vi "테승트.vi"() -> ()   [LabVIEW 2014]
uses:
  <vilib>/httpClient/LabVIEWHTTPClient.lvlib
panel:
  out "x fmc 플랜":string caption="본문"
  out "x fmc 다운로드 주소":string caption="화이트 스페이스가 제거된 문자열"
  out "trimmed string 4":string caption="화이트 스페이스가 제거된 문자열"
  out "body 2":string caption="본문"
  out "trimmed string 3":string caption="화이트 스페이스가 제거된 문자열"
  out "FMS  주소":string
  out "FMS 플랜":string caption="본문"
  out "trimmed string 2":string caption="화이트 스페이스가 제거된 문자열"
  out "trimmed string":string caption="화이트 스페이스가 제거된 문자열"
  in  "Destination":string
  in  "departure":string
  out "?":string
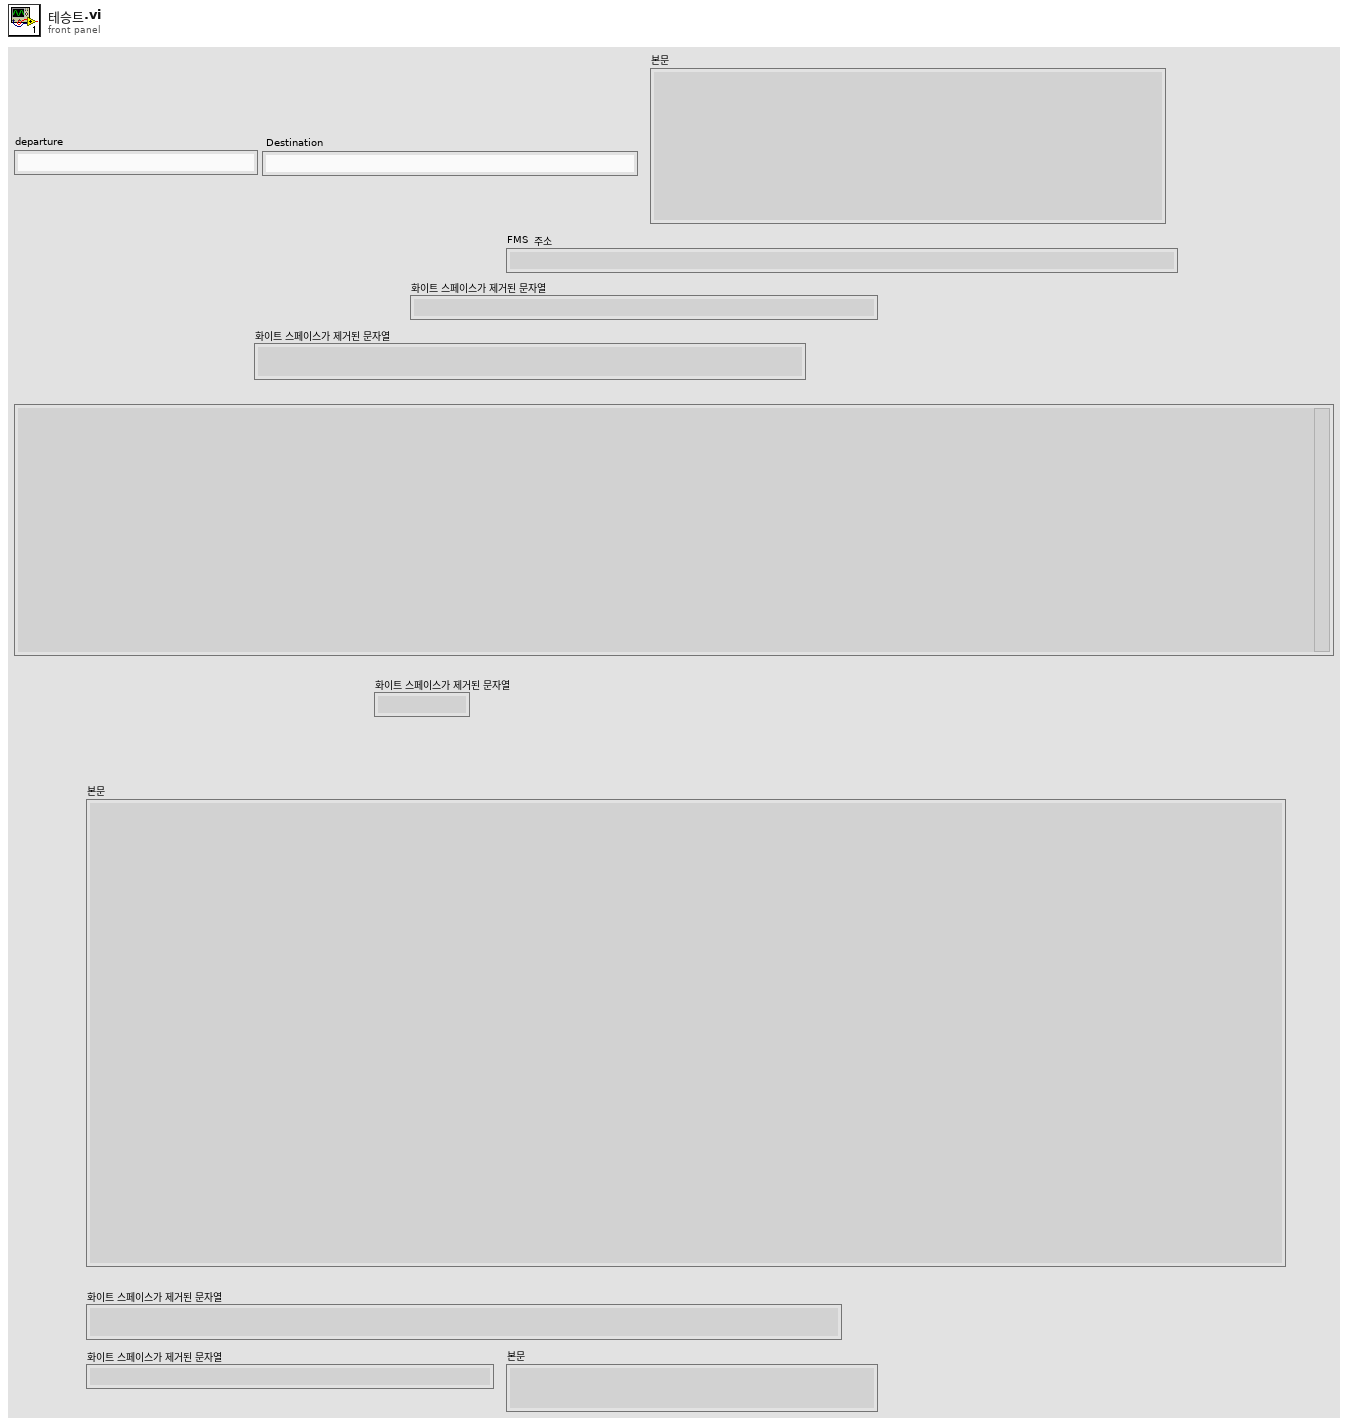
[diagram p1: front panel]
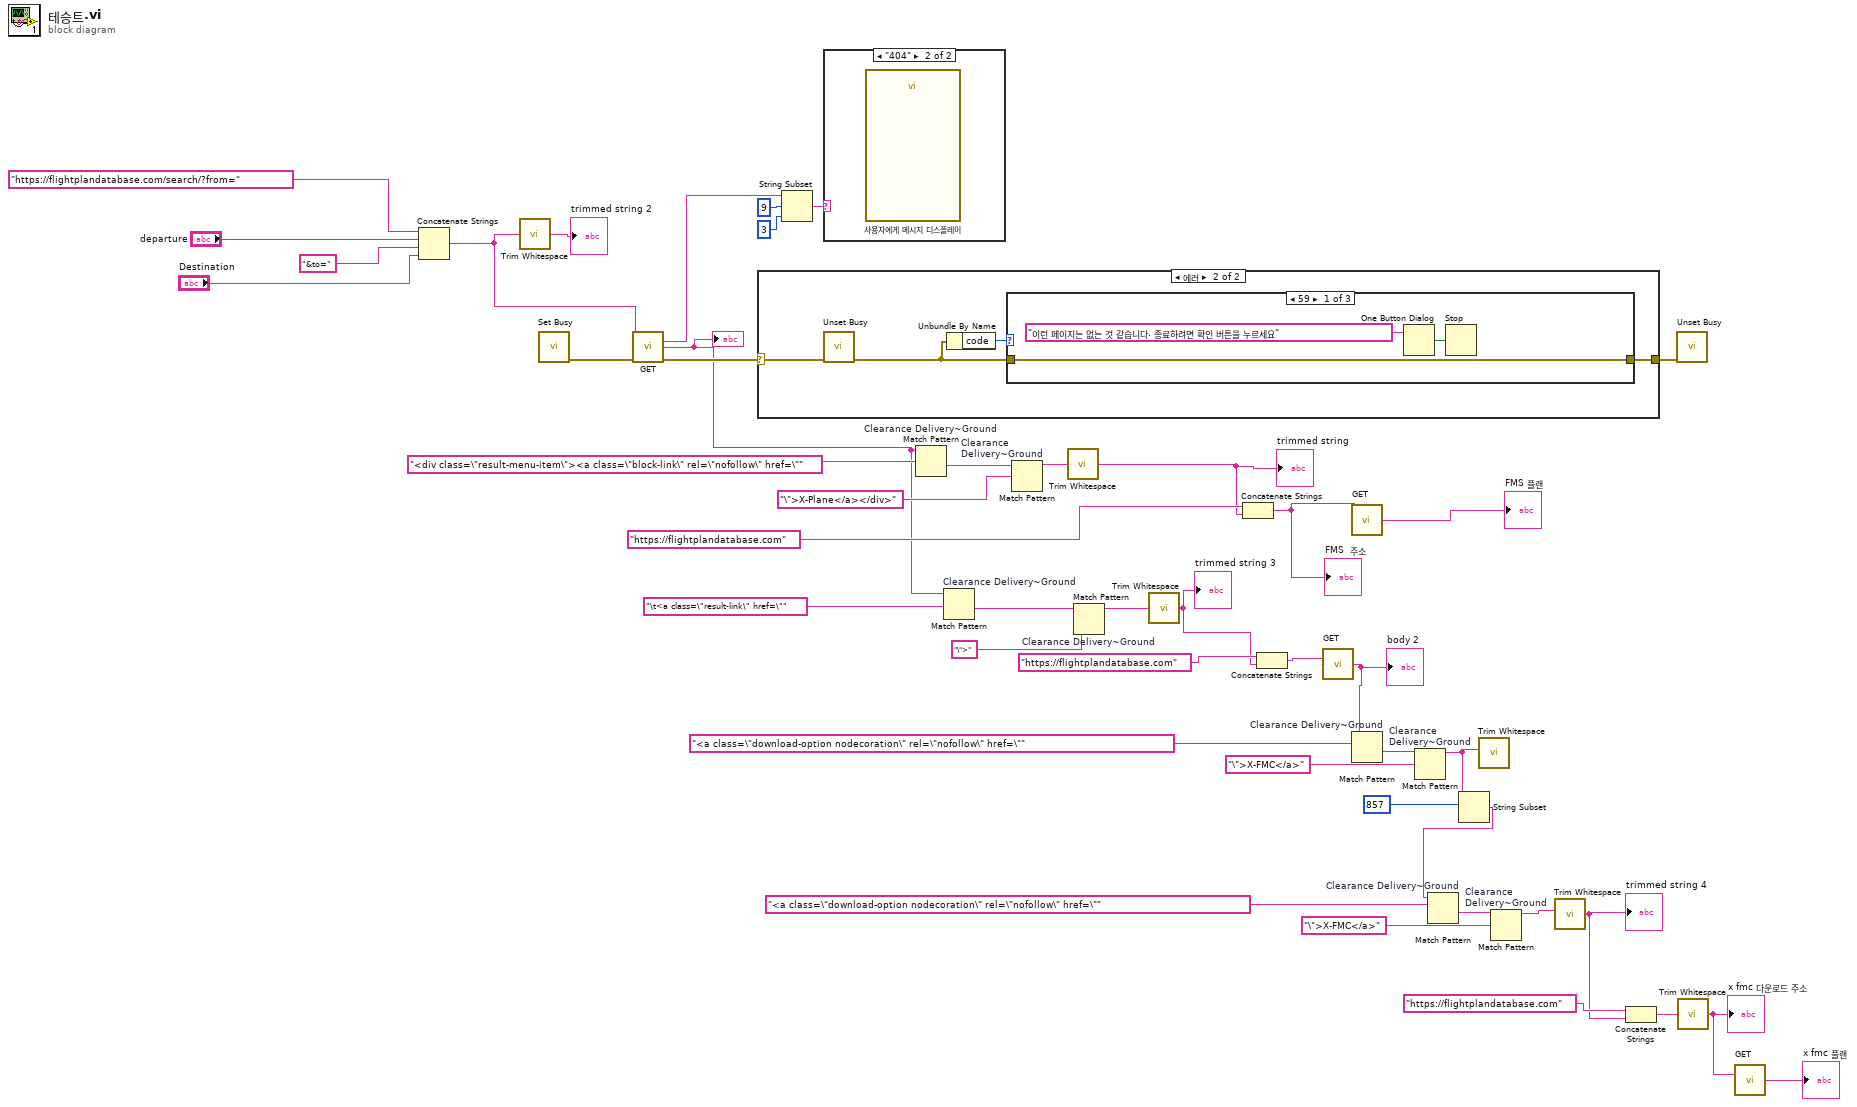
[diagram p0: block diagram]
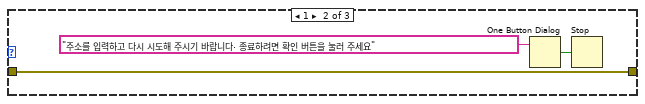
[diagram p4: hidden frame]
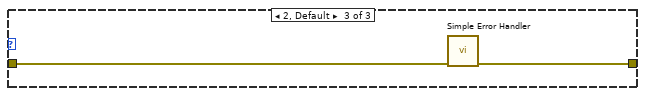
[diagram p5: hidden frame]
diagram:
  n1 = Concatenate Strings("https://flightplandatabase.com/search/?from=" ("문자열"), "departure", "&to=" ("문자열"), "Destination") -> (w32:string)
  n2 = call <vilib>:"Trim Whitespace.vi"("string"=w32) -> ("trimmed string"=→"trimmed string 2":string)  [unwired: 1 in]
  n3 = call <vilib>:"Set Busy.vi"() -> ("error out"=w40:errorcluster)  [unwired: 10 in, 1 out]
  n4 = call <vilib>:"GET.vi"("url"=w32, "error in (no error)"=w40) -> ("headers"=w44:string, "body"=w14:string, "error out"=w45:errorcluster)  [unwired: 10 in, 1 out]
  "?" <- w14
  n5 = case shown="에러" w45 {
    selector: w45 -> [w46 w49]
    tunnel: [w46 w47] -> w39
    frame No Error {
    }
    frame Error {
      n6 = call <vilib>:"Unset Busy.vi"("error in (no error)"=w49) -> ("error out"=w48:errorcluster)  [unwired: 10 in]
      n7 = Unbundle By Name(w48) -> ("code"=w50:i32)
      n8 = case shown="59" w50 {
        tunnel: w48 -> [w51 w56 w58]
        tunnel: [w51 w56 w57] -> w47
        frame 59 {
          n9 = One Button Dialog(message="이런 페이지는 없는 것 같습니다. 종료하려면 확인 버튼을 누르세요" ("메시지")) -> (true=w52:bool)  [unwired: 1 in]
          n10 = Stop(stop? (T)=w52) -> ()
        }
        frame 1 {
          n11 = One Button Dialog(message="주소를 입력하고 다시 시도해 주시기 바랍니다. 종료하려면 확인 버튼을 눌러 주세요" ("메시지")) -> (true=w54:bool)  [unwired: 1 in]
          n12 = Stop(stop? (T)=w54) -> ()
        }
        frame 2, Default {
          n13 = call <vilib>:"Simple Error Handler.vi"("error in (no error)"=w58) -> ("error out"=w57:errorcluster)  [unwired: 4 in, 4 out]
        }
      }
    }
  }
  n14 = String Subset(string=w44, offset (0)=9 ("오프셋(0)"), length (rest)=3 ("길이(나머지)")) -> (substring=w41:string)
  n15 = case shown="\"404\"" w41 {
    frame "거짓", Default {
    }
    frame "404" {
      n16 = call "사용자에게 메시지 디스플레이"() -> ()  [unwired: 10 in, 2 out]
    }
  }
  n17 = Match Pattern "Clearance Delivery~Ground"(string=w14, regular expression="<div class=\"result-menu-item\"><a class=\"block-link\" rel=\"nofollow\" href=\"" ("정규식")) -> (after substring=w35:string)  [unwired: 1 in, 3 out]
  n18 = Match Pattern "Clearance Delivery~Ground"(string=w14, regular expression="\t<a class=\"result-link\" href=\"" ("정규식")) -> (after substring=w24:string)  [unwired: 1 in, 3 out]
  n19 = Match Pattern "Clearance Delivery~Ground"(string=w35, regular expression="\">X-Plane</a></div>" ("정규식")) -> (before substring=w33:string)  [unwired: 1 in, 3 out]
  n20 = call <vilib>:"Trim Whitespace.vi"("string"=w33) -> ("trimmed string"=w26:string)  [unwired: 1 in]
  "trimmed string" <- w26
  n21 = Match Pattern "Clearance Delivery~Ground"(string=w24, regular expression="\">" ("정규식")) -> (before substring=w21:string)  [unwired: 1 in, 3 out]
  n22 = call <vilib>:"Trim Whitespace.vi"("string"=w21) -> ("trimmed string"=w19:string)  [unwired: 1 in]
  "trimmed string 3" <- w19
  n23 = Concatenate Strings("https://flightplandatabase.com" ("url"), w26) -> (w27:string)
  "FMS  주소" <- w27
  n24 = Concatenate Strings("https://flightplandatabase.com" ("url"), w19) -> (w16:string)
  n25 = call <vilib>:"GET.vi"("url"=w16) -> ("body"=w13:string)  [unwired: 11 in, 3 out]
  "body 2" <- w13
  n26 = call <vilib>:"GET.vi"("url"=w27) -> ("body"=→"FMS 플랜":string)  [unwired: 11 in, 3 out]
  n27 = Match Pattern "Clearance Delivery~Ground"(string=w13, regular expression="<a class=\"download-option nodecoration\" rel=\"nofollow\" href=\"" ("정규식")) -> (after substring=w15:string)  [unwired: 1 in, 3 out]
  n28 = Match Pattern "Clearance Delivery~Ground"(string=w15, regular expression="\">X-FMC</a>" ("정규식")) -> (before substring=w12:string)  [unwired: 1 in, 3 out]
  n29 = String Subset(string=w12, offset (0)=857 ("길이(나머지)")) -> (substring=w6:string)  [unwired: 1 in]
  n30 = Match Pattern "Clearance Delivery~Ground"(string=w6, regular expression="<a class=\"download-option nodecoration\" rel=\"nofollow\" href=\"" ("정규식")) -> (after substring=w8:string)  [unwired: 1 in, 3 out]
  n31 = call <vilib>:"Trim Whitespace.vi"("string"=w12) -> ()  [unwired: 1 in, 1 out]
  n32 = Match Pattern "Clearance Delivery~Ground"(string=w8, regular expression="\">X-FMC</a>" ("정규식")) -> (before substring=w7:string)  [unwired: 1 in, 3 out]
  n33 = call <vilib>:"Trim Whitespace.vi"("string"=w7) -> ("trimmed string"=w4:string)  [unwired: 1 in]
  "trimmed string 4" <- w4
  n34 = Concatenate Strings("https://flightplandatabase.com" ("url"), w4) -> (w3:string)
  n35 = call <vilib>:"Unset Busy.vi"("error in (no error)"=w39) -> ()  [unwired: 10 in, 1 out]
  n36 = call <vilib>:"Trim Whitespace.vi"("string"=w3) -> ("trimmed string"=w2:string)  [unwired: 1 in]
  "x fmc 다운로드 주소" <- w2
  n37 = call <vilib>:"GET.vi"("url"=w2) -> ("body"=→"x fmc 플랜":string)  [unwired: 11 in, 3 out]
